vi "RenameMessage.vi"(8 "error in (no error)":errorcluster, 10 "Message Name":string, 11 "Message in":refnum<class "Message.lvclass">) -> (0 "error out":errorcluster, 3 "Message out":refnum<class "Message.lvclass">)   [LabVIEW 2009, in "LapDog.Messaging.v2.lvlib" / "Message.lvclass"]
doc: "Changes the name of a message object. If an empty string is connected to the Message Name terminal, Get MessageName will return the name of the class.\n\nThis method executes regardless of the error in state."
uses:
  Message.lvclass
  Message.lvclass/Message.ctl
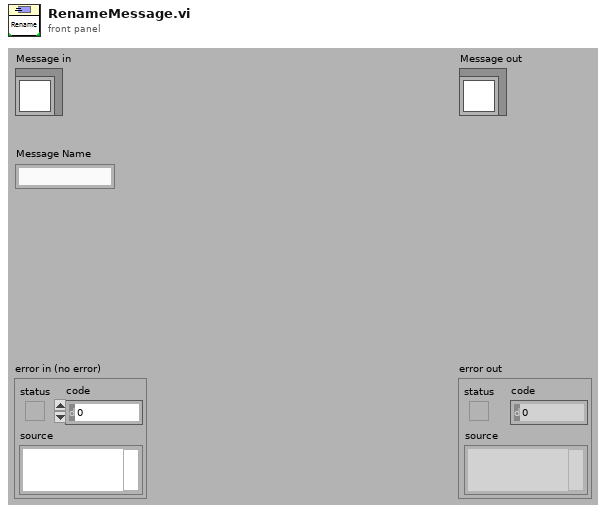
[diagram p1: front panel]
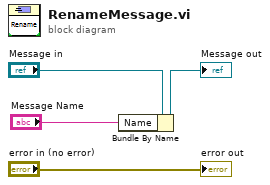
[diagram p0: block diagram]
diagram:
  n1 = Bundle By Name(cluster="Message in", "Name"="Message Name") -> (→"Message out":refnum<class "Message.lvclass">)
  "error out" <- "error in (no error)"
